vi "HRR-IntelRead.vi"(8 "error in (no error)":errorcluster, 10 "Intel in":u8, 11 "VISA resource name in":refnum<visa-resource-name>) -> (0 "error out":errorcluster, 2 "Intel out":u8, 3 "VISA resource name out":refnum<visa-resource-name>)   [LabVIEW 2019]
panel:
  out "Bytes at Port":u32
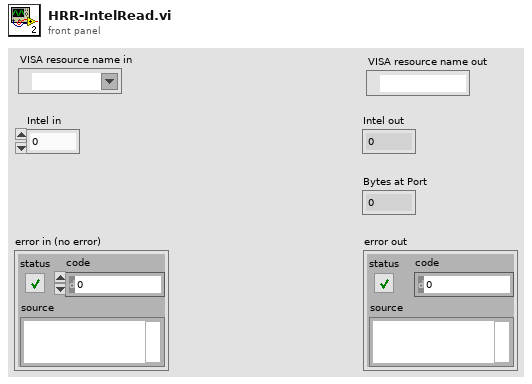
[diagram p1: front panel]
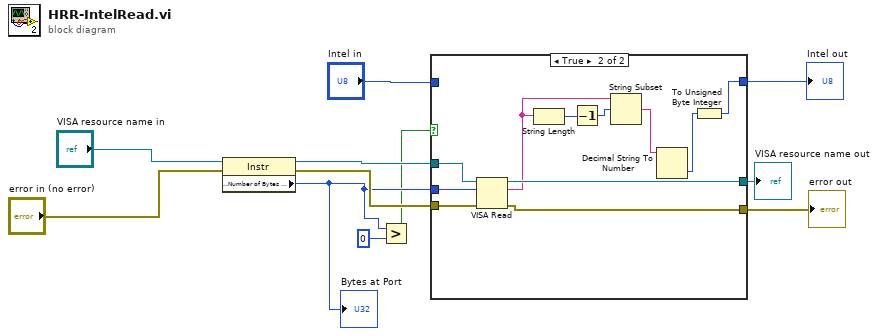
[diagram p0: block diagram]
diagram:
  n1 = property class="Instr"(reference="VISA resource name in", error in="error in (no error)") -> (reference out=w11:refnum<visa-resource-name>, error out=w9:errorcluster, "Serial Settings:Number of Bytes at Serial Port"=w8:u32)
  "Bytes at Port" <- w8
  n2 = Greater?(x=w8, y=u32 0) -> (0:w6:bool)
  n3 = case shown="True" w6 {
    tunnel: w8 -> [_ w25]
    tunnel: w11 -> [w13 w24]
    tunnel: w9 -> [w14 w23]
    tunnel: [w14 w22] -> w5
    tunnel: [w12 w20] -> w2
    tunnel: [w13 w19] -> w3
    tunnel: "Intel in" -> [w12 _]
    frame False {
    }
    frame True {
      n4 = VISA Read(VISA resource name=w24, byte count=w25, error in (no error)=w23) -> (VISA resource name out=w19:refnum<visa-resource-name>, read buffer=w16:string, error out=w22:errorcluster)  [unwired: 1 out]
      n5 = String Length(string=w16) -> (length=w18:i32)
      n6 = Decrement(x=w18) -> (x-1=w17:i32)
      n7 = String Subset(string=w16, offset (0)=w17) -> (substring=w15:string)  [unwired: 1 in]
      n8 = Decimal String To Number(string=w15) -> (number=w21:i32)  [unwired: 2 in, 1 out]
      n9 = To Unsigned Byte Integer(number=w21) -> (unsigned 8bit integer=w20:u8)
    }
  }
  "error out" <- w5
  "Intel out" <- w2
  "VISA resource name out" <- w3
